vi "Is Materials Enough to Build a Robot.vi"(1 "Inventory":T1, 2 "Robot Building Cost":T2[](array[typedef]) {"Mineral" items=["Ore", "Clay", "Obsidian", "Geode", "Open Geode"]}) -> (3 "Is Materials Enough to Build a Robot ?":bool)   [LabVIEW 2020, in "AoC 2022.lvlib"]
uses:
  AoC 2022.lvlib
  Mineral_Enum.ctl
  Mineral.ctl
  Cost.ctl
  Inventory.ctl
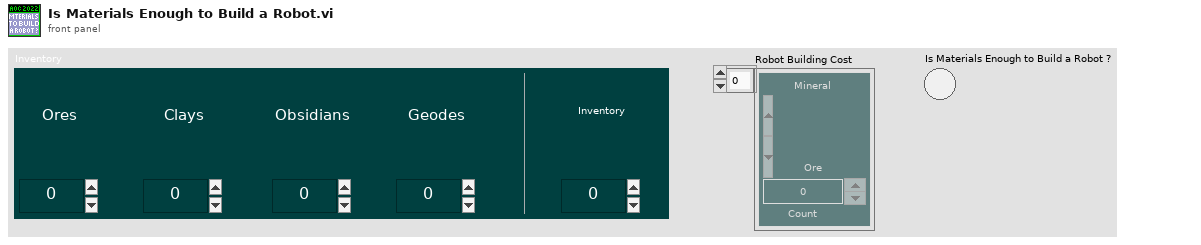
[diagram p1: front panel]
types:
  T1 = typedef "AoC 2022.lvlib/Inventory.ctl" = cluster{"Ores":u32, "Clays":u32, "Obsidians":u32, "Geodes":u32, "Inventory":u32}
  T2 = typedef "AoC 2022.lvlib/Cost.ctl" = cluster{"Mineral":T3, "Count":u32}
  T3 = typedef "AoC 2022.lvlib/Mineral.ctl" = u16
  T4 = typedef "AoC 2022.lvlib/Mineral_Enum.ctl" = enum16{"ore", "clay", "obsidian", "geode", "Open Geode"}
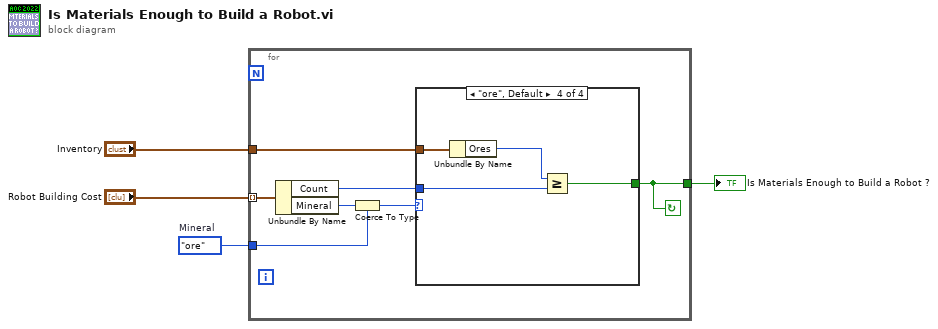
[diagram p0: block diagram]
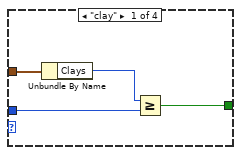
[diagram p2: hidden frame]
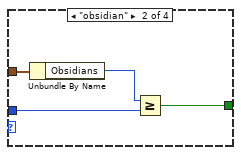
[diagram p3: hidden frame]
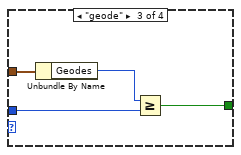
[diagram p4: hidden frame]
diagram:
  w1 = Mineral_Enum."ore"  # Mineral
  n1 = for {
    tunnel: "Robot Building Cost" -> [w11] mode=indexing
    tunnel: "Inventory" -> [w8]
    tunnel: [w6] -> w3
    tunnel: w1 -> [w5]
    stop <- w6 continue-if-true
    n2 = Unbundle By Name(w11) -> ("Count"=w7:u32, "Mineral"=w10:T3)
    n3 = Coerce To Type(0:w10, 1:w5) -> (2:w9:T4)
    n4 = case shown="\"ore\", Default" w9 {
      tunnel: w8 -> [w15 w19 w23 w27]
      tunnel: w7 -> [w13 w17 w21 w25]
      tunnel: [w12 w16 w20 w24] -> w6
      frame "clay" {
        n5 = Unbundle By Name(w15) -> ("Clays"=w14:u32)
        n6 = Greater Or Equal?(x=w14, y=w13) -> (x >= y?=w12:bool)
      }
      frame "obsidian" {
        n7 = Unbundle By Name(w19) -> ("Obsidians"=w18:u32)
        n8 = Greater Or Equal?(x=w18, y=w17) -> (x >= y?=w16:bool)
      }
      frame "geode" {
        n9 = Unbundle By Name(w23) -> ("Geodes"=w22:u32)
        n10 = Greater Or Equal?(x=w22, y=w21) -> (x >= y?=w20:bool)
      }
      frame "ore", Default {
        n11 = Unbundle By Name(w27) -> ("Ores"=w26:u32)
        n12 = Greater Or Equal?(x=w26, y=w25) -> (x >= y?=w24:bool)
      }
    }
  }
  "Is Materials Enough to Build a Robot ?" <- w3
